vi "BuckConverterWeb.vi"(7 "LabVIEW Web Service Request":refnum<class "Web Request.lvclass">) -> ()   [LabVIEW 2015]
uses:
  <vilib>/wsapi/Web Request.lvclass
  <vilib>/imath/engines/lvmath2/RunTimeEngine/Managers/WorkSpace/UID Generator.vi
  <vilib>/imath/engines/lvmath/Plug In/Control Design/BuiltInFunctions/tf/NIMS_CD_tf(STR,Ts).vi
  <vilib>/imathl/engines/lvmath/Functions/Error Handling/Create Error.vi
  <vilib>/imath/engines/lvmath/Plug In/Control Design/BuiltInFunctions/multmx/NIMS_CD_multmx(TF,K).vi
  <vilib>/imath/engines/lvmath/Plug In/Control Design/BuiltInFunctions/plus/NIMS_CD_plus(K,TF).vi
  <vilib>/imath/engines/lvmath/Functions/Error Handling/MergeErrorsWrapper.vi
  <vilib>/imath/engines/lvmath/Plug In/Control Design/BuiltInFunctions/powermx/NIMS_CD_powermx(TF,N).vi
  <vilib>/imath/engines/lvmath/Plug In/Control Design/BuiltInFunctions/plus/NIMS_CD_plus(TF,TF).vi
  <vilib>/imath/engines/lvmath/Plug In/Control Design/BuiltInFunctions/rightdivmx/NIMS_CD_rightdivmx(TF,TF).vi
  <vilib>/imath/engines/lvmath2/RunTimeEngine/RunTimeType/NIMS_RunTimeType_From StrictType (excl LVString).vi
  <instcachedir>/0/NIMS_RunTimeType_From StrictType (excl LVString)_EB1C38A9BC5048DA9ABDA8F781E54D21.lvgen/NIMS_RunTimeType_From StrictType (excl LVString)_EB1C38A9BC5048DA9ABDA8F781E54D21_031.vi
  <vilib>/imath/engines/lvmath2/RunTimeEngine/LocalVariableDefStatement/MC_LocalVariableDefStatement_Display.vi
  <vilib>/imath/engines/lvmath/Plug In/Control Design/BuiltInFunctions/multmx/NIMS_CD_multmx(K,TF).vi
  <vilib>/imath/engines/lvmath/Plug In/Control Design/BuiltInFunctions/step/NIMS_CD_[Y,T]=step(TF,[Tinfo]).vi
  <vilib>/imath/engines/lvmath2/RunTimeEngine/Managers/SymbolTable/Clear UID.vi
  <vilib>/imath/engines/lvmath2/RunTimeEngine/NodeEndStatement/NIMS_NodeEndStatement_Output.vi
  <instcachedir>/0/NIMS_NodeEndStatement_Output_53EC0D466D134D7ABD903AC30B43404B.lvgen/NIMS_NodeEndStatement_Output_53EC0D466D134D7ABD903AC30B43404B_001.vi
  <vilib>/imath/engines/lvmath2/RunTimeEngine/ErrorHandling/NIMS_Finalize Error.vi
  <vilib>/imath/engines/lvmath2/RunTimeEngine/Managers/SymbolTable/NIMS_WorkSpace.lvlib
panel:
  out "error out":errorcluster
  out "JSON string":string
  in  "error in (no error)":errorcluster
  # "Use the Web Service Request input terminal to call the VIs on the Web Services palette. Do not remove it from the connector pane unless you don't need access to the palette."
  # "Each additional control wired to the connector pane will be available as an input in the URL. To include an indicator in terminal-mode output (the default setting), it must also be wired to the connector pane."
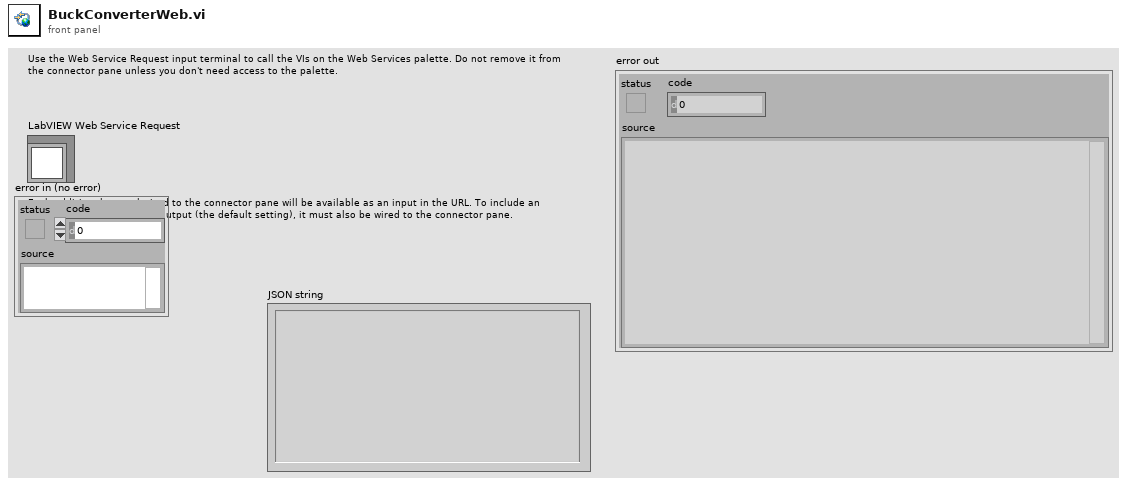
[diagram p1: front panel]
types:
  T1 = cluster{"Vo":dbl, "Io":dbl, "P":dbl, "deltaIL":dbl}
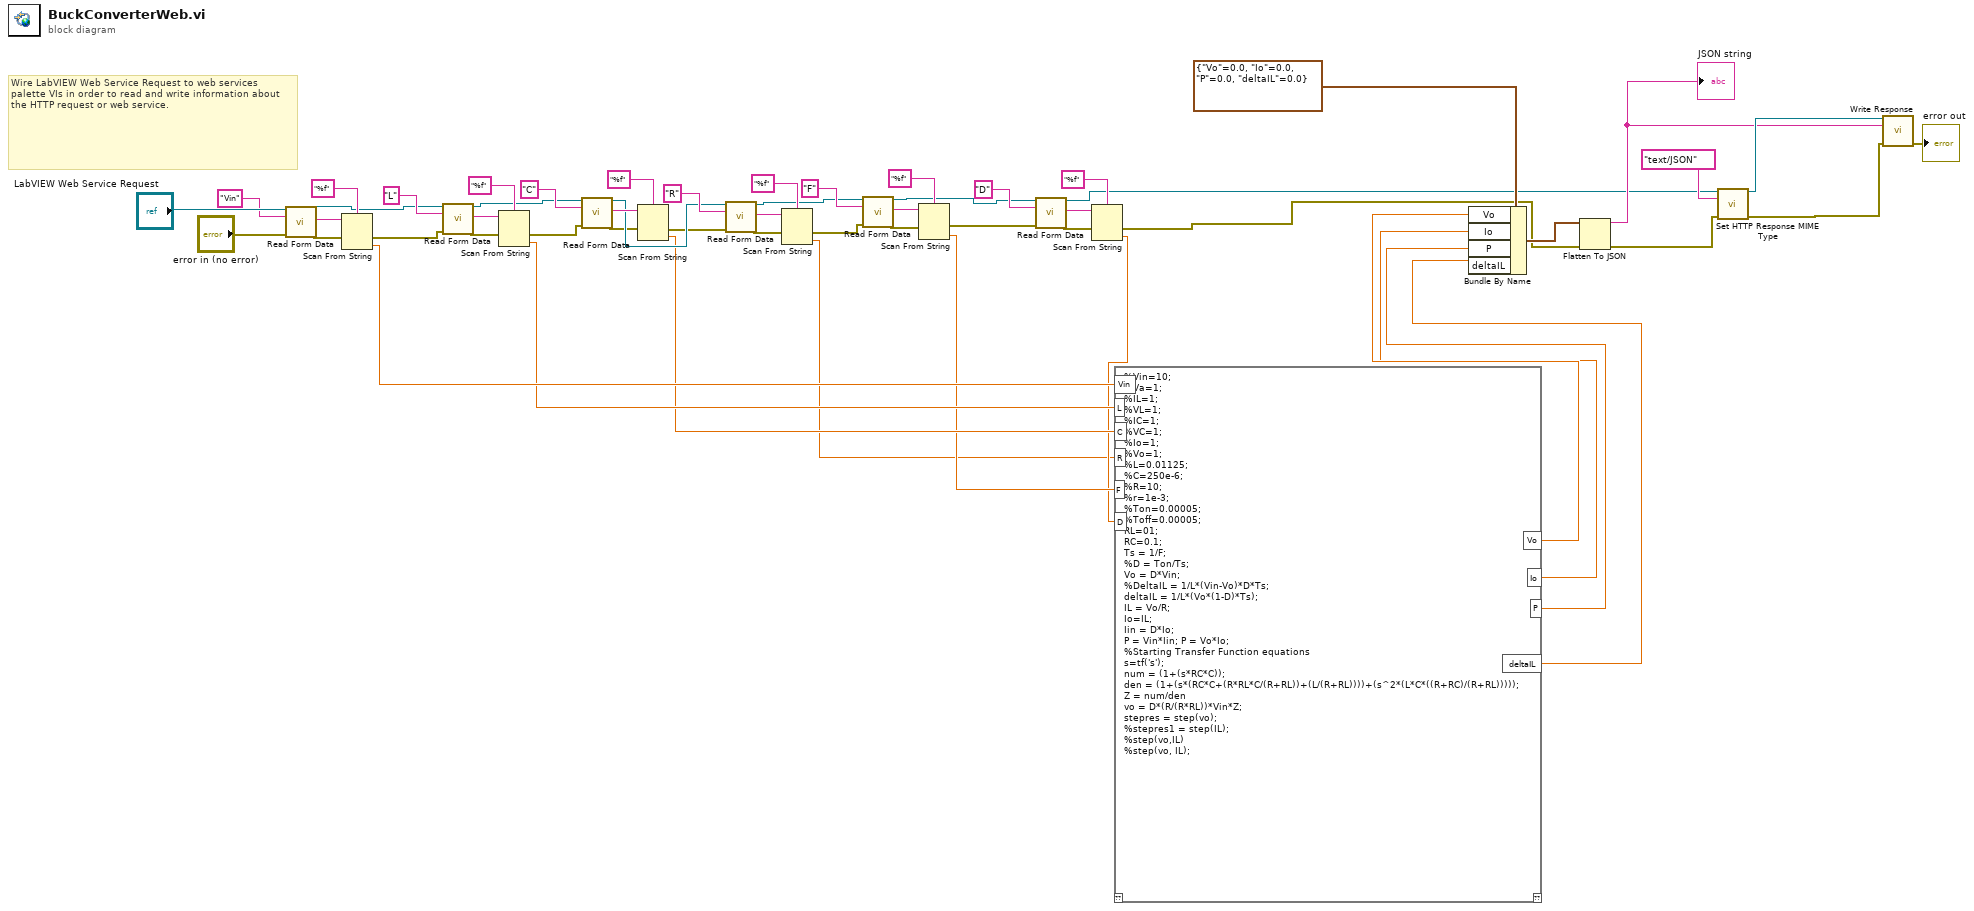
[diagram p0: block diagram]
diagram:
  # "Wire LabVIEW Web Service Request to web services palette VIs in order to read and write information about the HTTP request or web service."
  n1 = call <vilib>:"Read Form Data.vi"("LabVIEW Web Service Request"="LabVIEW Web Service Request", "key"="Vin", "error in (no error)"="error in (no error)") -> ("LabVIEW Web Service Request out"=w50:refnum<class "Web Request.lvclass">, "value"=w53:string, "error out"=w20:errorcluster)  [unwired: 9 in, 1 out]
  n2 = Scan From String(format string="%f", input string=w53, error in=w20) -> (error out=w21:errorcluster, output 1=w18:dbl)  [unwired: 2 in, 2 out]
  n3 = call <vilib>:"Read Form Data.vi"("LabVIEW Web Service Request"=w50, "key"="L", "error in (no error)"=w21) -> ("LabVIEW Web Service Request out"=w45:refnum<class "Web Request.lvclass">, "value"=w51:string, "error out"=w22:errorcluster)  [unwired: 9 in, 1 out]
  n4 = Scan From String(format string="%f", input string=w51, error in=w22) -> (error out=w23:errorcluster, output 1=w17:dbl)  [unwired: 2 in, 2 out]
  n5 = call <vilib>:"Read Form Data.vi"("LabVIEW Web Service Request"=w45, "key"="C", "error in (no error)"=w23) -> ("LabVIEW Web Service Request out"=w41:refnum<class "Web Request.lvclass">, "value"=w47:string, "error out"=w24:errorcluster)  [unwired: 9 in, 1 out]
  n6 = Scan From String(format string="%f", input string=w47, error in=w24) -> (error out=w25:errorcluster, output 1=w16:dbl)  [unwired: 2 in, 2 out]
  n7 = call <vilib>:"Read Form Data.vi"("LabVIEW Web Service Request"=w41, "key"="R", "error in (no error)"=w25) -> ("LabVIEW Web Service Request out"=w37:refnum<class "Web Request.lvclass">, "value"=w43:string, "error out"=w26:errorcluster)  [unwired: 9 in, 1 out]
  n8 = Scan From String(format string="%f", input string=w43, error in=w26) -> (error out=w27:errorcluster, output 1=w6:dbl)  [unwired: 2 in, 2 out]
  n9 = call <vilib>:"Read Form Data.vi"("LabVIEW Web Service Request"=w37, "key"="F", "error in (no error)"=w27) -> ("LabVIEW Web Service Request out"=w33:refnum<class "Web Request.lvclass">, "value"=w39:string, "error out"=w28:errorcluster)  [unwired: 9 in, 1 out]
  n10 = Scan From String(format string="%f", input string=w39, error in=w28) -> (error out=w29:errorcluster, output 1=w15:dbl)  [unwired: 2 in, 2 out]
  n11 = call <vilib>:"Read Form Data.vi"("LabVIEW Web Service Request"=w33, "key"="D", "error in (no error)"=w29) -> ("LabVIEW Web Service Request out"=w2:refnum<class "Web Request.lvclass">, "value"=w35:string, "error out"=w30:errorcluster)  [unwired: 9 in, 1 out]
  n12 = Scan From String(format string="%f", input string=w35, error in=w30) -> (error out=w1:errorcluster, output 1=w14:dbl)  [unwired: 2 in, 2 out]
  n13 = mathscript code="%Vin=10;\n%Va=1;\n%IL=1;\n%VL=1;\n%IC=1;\n%VC=1;\n%Io=1;\n%Vo=1;\n%L=0.01125;\n%C=250e-6;\n%R=10;\n%r=1e-3;\n%Ton=0.00005;\n%Toff=0.00005;\nRL=01;\nRC=0.1;\nTs = 1/F;\n%D = Ton/Ts;\nVo = D*Vin;\n%DeltaIL = 1/L*(Vin-Vo)*D*Ts;\ndeltaIL = 1/L*(Vo*(1-D)*Ts);\nIL = Vo/R;\nIo=IL;\nIin = D*Io;\nP = Vin*Iin; P = Vo*Io;\n%Starting Transfer Function equations\ns=tf('s');\nnum = (1+(s*RC*C));\nden = (1+(s*(RC*C+(R*RL*C/(R+RL))+(L/(R+RL))))+(s^2*(L*C*((R+RC)/(R+RL)))));\nZ = num/den\nvo = D*(R/(R*RL))*Vin*Z;\nstepres = step(vo);\n%stepres1 = step(IL);\n%step(vo,IL)\n%step(vo, IL);"("Vin"=w18, "L"=w17, "C"=w16, "R"=w6, "F"=w15, "D"=w14) -> ("Vo"=w13:dbl, "Io"=w7:dbl, "P"=w12:dbl, "deltaIL"=w11:dbl)  [unwired: 1 in, 1 out]
  n14 = Bundle By Name(cluster=T1 {"Vo"=0.0, "Io"=0.0, "P"=0.0, "deltaIL"=0.0} ("input cluster"), "Vo"=w13, "Io"=w7, "P"=w12, "deltaIL"=w11) -> (w5:T1)
  n15 = Flatten To JSON(anything=w5, error in (no error)=w1) -> (JSON string=w4:string, 11:w3:errorcluster)  [unwired: 1 in]
  "JSON string" <- w4
  n16 = call <vilib>:"Set HTTP Response MIME Type.vi"("LabVIEW Web Service Request"=w2, "MIME type (text/html)"="text/JSON", "error in (no error)"=w3) -> ("LabVIEW Web Service Request out"=w10:refnum<class "Web Request.lvclass">, "error out"=w9:errorcluster)  [unwired: 11 in]
  n17 = call <vilib>:"Write Response.vi"("LabVIEW Web Service Request"=w10, "response string"=w4, "error in (no error)"=w9) -> ("error out"=→"error out":errorcluster)  [unwired: 11 in, 1 out]
